vi "Vector Unique Values String.vi"(1 "array in":string[](array[string])) -> (0 "uniques out":string[](array[string]))   [LabVIEW 2020]
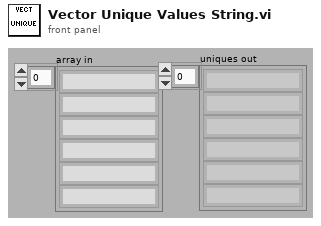
[diagram p1: front panel]
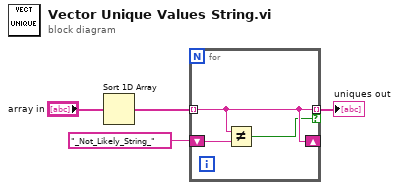
[diagram p0: block diagram]
diagram:
  n1 = Sort 1D Array(array="array in") -> (sorted array=w3:string[])
  n2 = for {
    tunnel: w3 -> [w6] mode=indexing
    shift-right: [w6] -> _
    shift-left: "_Not_Likely_String_" -> [w7]
    tunnel: [w6] -> w2 mode=indexing if=w5
    n3 = Not Equal?(x=w6, y=w7) -> (x != y?=w5:bool)
  }
  "uniques out" <- w2
